vi "In V.vi"(9 "VISA resource name":refnum<visa-resource-name>="com4", 10 "升温速度":string) -> ()   [LabVIEW 2021]
uses:
  <vilib>/Instr/_visa.llb/VISA Configure Serial Port (Instr).vi
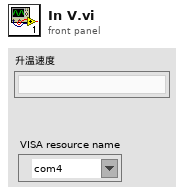
[diagram p1: front panel]
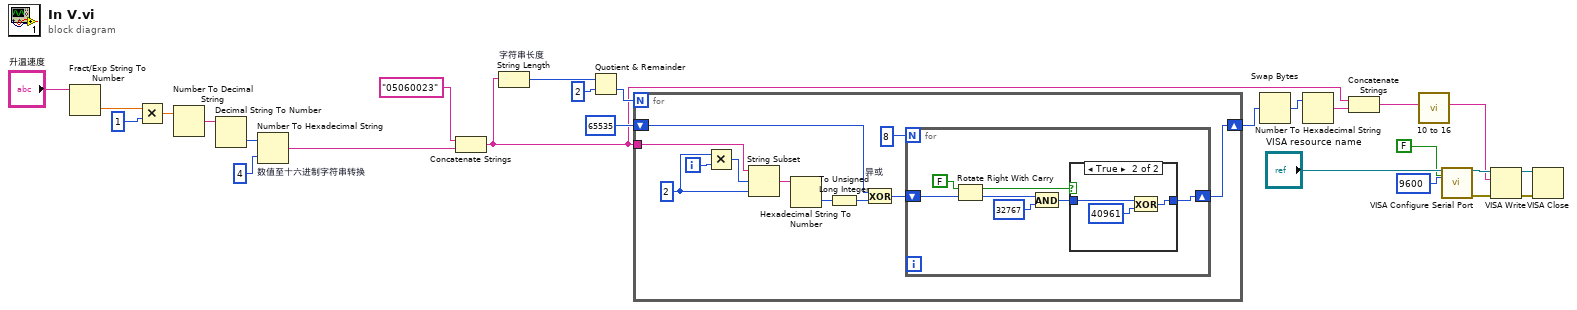
[diagram p0: block diagram]
diagram:
  n1 = Fract/Exp String To Number(string="升温速度") -> (number=w4:dbl)  [unwired: 3 in, 1 out]
  n2 = Multiply(x=w4, y=1) -> (x*y=w3:dbl)
  n3 = Number To Decimal String(number=w3) -> (decimal integer string=w2:string)  [unwired: 1 in]
  n4 = Decimal String To Number(string=w2) -> (number=w23:i32)  [unwired: 2 in, 1 out]
  n5 = Number To Hexadecimal String "数值至十六进制字符串转换"(1:4, 2:w23) -> (0:w24:string)
  n6 = Concatenate Strings("05060023" ("写入缓冲区"), w24) -> (w15:string)
  n7 = String Length "字符串长度"(string=w15) -> (length=w20:i32)
  n8 = Quotient & Remainder(x=w20, y=2) -> (floor(x/y)=w22:i32)  [unwired: 1 out]
  n9 = for {
    N: w22 -> [_]
    tunnel: w15 -> [w37]
    shift-right: [w27] -> w18
    shift-left: 65535 -> [w28]
    i -> [w35]
    w36 = 2
    n10 = Multiply(x=w36, y=w35) -> (x*y=w34:i32)
    n11 = String Subset ("截取字符串")(string=w37, offset (0)=w34, length (rest)=w36) -> (substring=w33:string)
    n12 = Hexadecimal String To Number ("十六进制数字符串至数值转换")(string=w33) -> (number=w32:u32)  [unwired: 2 in, 1 out]
    n13 = To Unsigned Long Integer ("转换为无符号长整型")(number=w32) -> (unsigned 32bit integer=w31:u32)
    n14 = Exclusive Or "异或"(1:w31, 2:w28) -> (0:w29:u32)
    n15 = for {
      N: 8 -> [_]
      shift-right: [w42] -> w27
      shift-left: w29 -> [w44]
      n16 = Rotate Right With Carry(2:w44, 3:FALSE) -> (0:w40:u32, 1:w41:bool)
      n17 = And(x=w40, y=u32 32767) -> (x .and. y?=w39:u32)
      n18 = case shown="True" w41 {
        tunnel: w39 -> [w45 w47]
        tunnel: [w45 w46] -> w42
        frame False {
        }
        frame True {
          n19 = Exclusive Or(1:u32 40961, 2:w47) -> (0:w46:u32)
        }
      }
    }
  }
  n20 = Swap Bytes ("交换字节")(anything=w18) -> (byte swapped=w17:u32)
  n21 = Number To Hexadecimal String ("数值至十六进制字符串转换")(2:w17) -> (0:w16:string)  [unwired: 1 in]
  n22 = Concatenate Strings(w15, w16) -> (w8:string)
  n23 = call "10 to 16.vi"("字符串"=w8) -> ("字符串 2"=w7:string)  [unwired: 10 in]
  n24 = call-poly "VISA Configure Serial Port"("VISA resource name"="VISA resource name", "Enable Termination\nChar (T)"=FALSE ("确定按钮"), "baud rate (9600)"=u32 9600) -> ("VISA resource name out"=w13:refnum<visa-resource-name>, "error out"=w9:errorcluster)  [unwired: 11 in]
  n25 = VISA Write ("VISA写入")(VISA resource name=w13, write buffer=w7, error in (no error)=w9) -> (VISA resource name out=w11:refnum<visa-resource-name>, error out=w10:errorcluster)  [unwired: 1 out]
  n26 = VISA Close(VISA resource name=w11, error in (no error)=w10) -> ()  [unwired: 1 out]
